vi "SpinnyInitMotor.vi"(8 "error in":errorcluster) -> (0 "error out":errorcluster, 3 "Arduino Resource Out":T1={"VISA resource"="", "Board Type"=enum."Uno", "Connection Type"=enum."USB / Serial", "Bytes Per Packet (15)"=15})   [LabVIEW 2014]
uses:
  <vilib>/LabVIEW Interface for Arduino/Type Defs/Arduino Resource.ctl
  <vilib>/LabVIEW Interface for Arduino/Type Defs/Board Type.ctl
  <vilib>/LabVIEW Interface for Arduino/LabVIEW Interface for Arduino.lvlib
panel:
  in  "Stepper #":u8=1
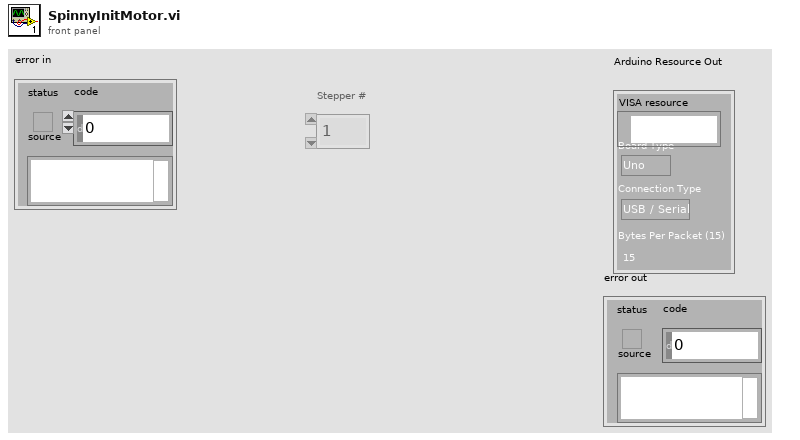
[diagram p1: front panel]
types:
  T1 = typedef "LabVIEW Interface for Arduino.lvlib/Arduino Resource.ctl" = cluster{"VISA resource":refnum<visa-resource-name>, "Board Type":T2, "Connection Type":enum8{"USB / Serial"}, "Bytes Per Packet (15)":u8}
  T2 = typedef "LabVIEW Interface for Arduino.lvlib/Board Type.ctl" = enum16{"Uno", "Dimuelanove w/Atmega 328", "Mega 2560"}
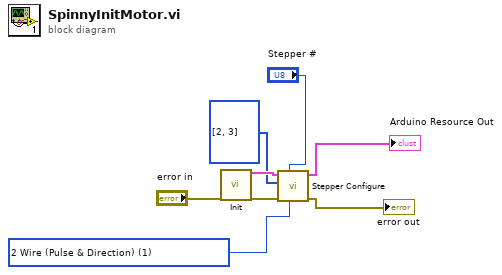
[diagram p0: block diagram]
diagram:
  w5 = u8 1 items=["2 Wire (Pulse & Direction)"=1, "2 Wire"=2, "4 Wire"=4, "EasyDriver"=6, "AF Motor Shield (Stepper 1 & 2 Only)"=5] ("Control Method")
  n1 = call <vilib>:"Init.vi"("error in"="error in") -> ("Arduino Resource"=w8:T1, "error out"=w7:errorcluster)  [unwired: 17 in]
  n2 = call <vilib>:"Stepper Configure.vi"("Control Method"=w5, "Stepper #"="Stepper #", "error in"=w7, "Stepper Pins"=u8[] [2, 3], "Arduino Resource"=w8) -> ("error out"=→"error out":errorcluster, "Arduino Resource Out"=→"Arduino Resource Out":T1)  [unwired: 5 in]
